vi "Reference 2 Pointer.vi"(0 "Generic Reference":refnum<data-value>) -> (1 "Valid?":bool, 2 "Pointer":u64 format="%.0x")   [LabVIEW 2013, in "Hierarchy Framework.lvlib" / "Generic.lvclass"]
uses:
  Generic.lvclass
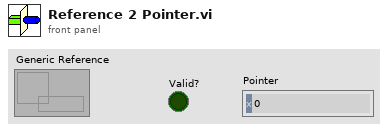
[diagram p1: front panel]
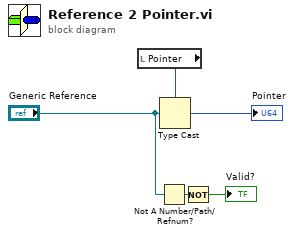
[diagram p0: block diagram]
diagram:
  n1 = local read "Pointer"() -> (w5:u64)
  n2 = Not A Number/Path/Refnum?(number/path/refnum="Generic Reference") -> (NaN/Path/Refnum?=w3:bool)
  n3 = Type Cast(type=w5, x="Generic Reference") -> (*(type *) &x=→"Pointer":u64)
  n4 = Not(x=w3) -> (.not. x?=→"Valid?":bool)
